vi "Windows.vi"(2 "Tau":dbl[](array[numeric]) format="%.3f", 3 "WINDOW":u16(ring) items=["FlatTop1", "FlatTop2", "FlatTop3", "FlatTop4", "FlatTop5", "FlatTop6"]) -> (0 "dPsi":dbl[](array[numeric]) format="%.3g", 1 "Psi":dbl[](array[numeric]) format="%.3g")   [LabVIEW 2022 SP3]
uses:
  <vilib>/Utility/file.llb/Read From Spreadsheet File (DBL).vi
  <vilib>/express/express arith-compare/Formula/XNode/ExpressFormulaBlockNode.xnode
panel:
  in  "ROWS":dbl
  in  "NEURONS":dbl
  in  "COLS":dbl
  in  "K":dbl
  out "DERIVATE FlatTop":dbl[][](array[numeric])
  out "FUNCTION FlatTop":dbl[][](array[numeric])
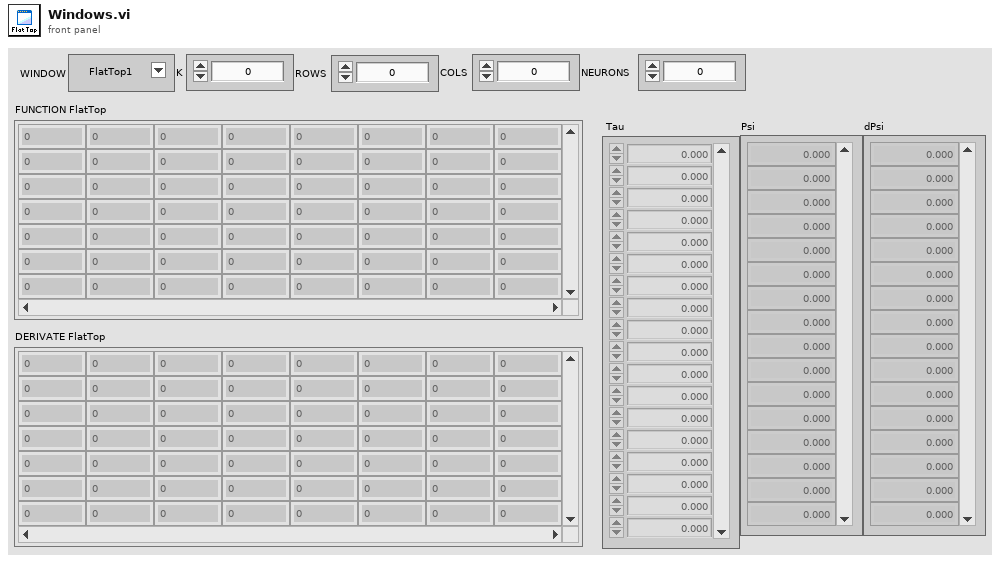
[diagram p1: front panel]
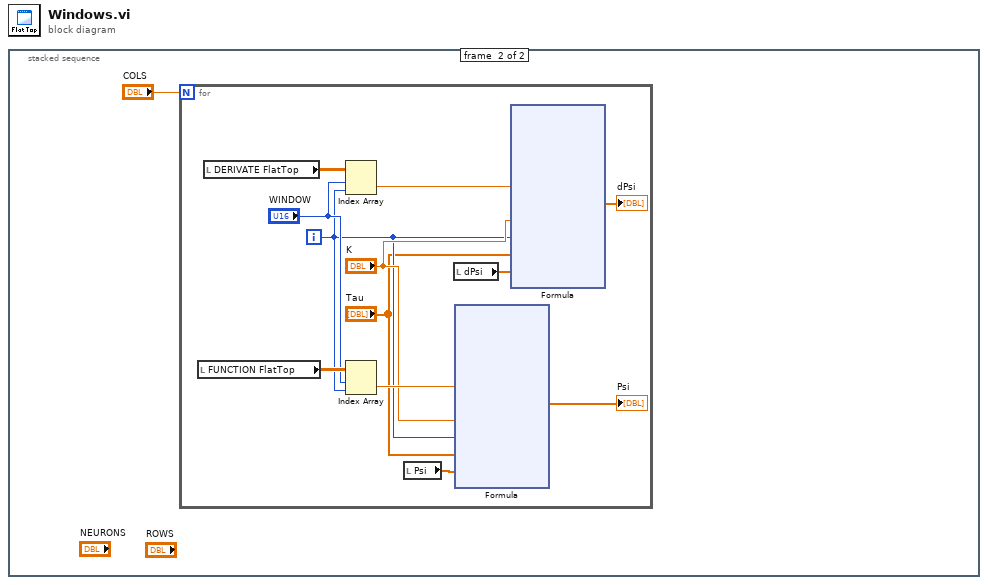
[diagram p0: block diagram]
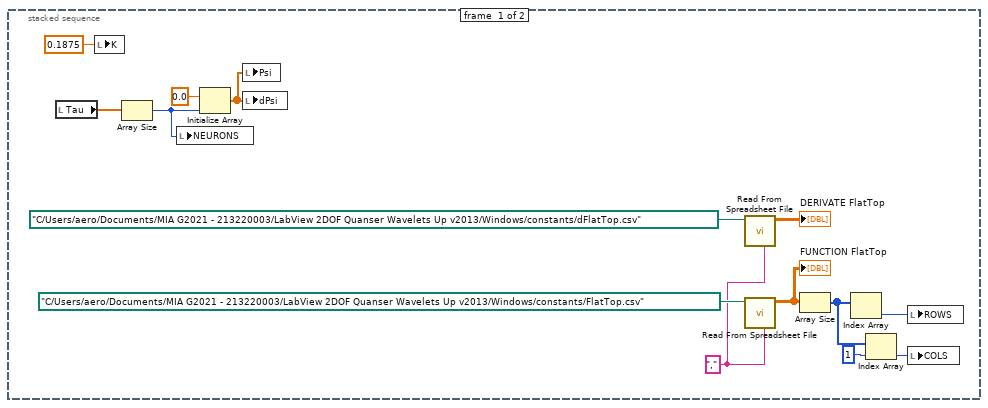
[diagram p2: hidden frame]
diagram:
  n1 = stacked-sequence {
    frame #0 {
      w2 = "," ("delimiter (\\t)")
      n2 = local read "Tau"() -> (w9:dbl[])
      n3 = local write "K"(0.1875 ("K")) -> ()
      n4 = Array Size(array=w9) -> (size(s)=w7:i32)
      n5 = local write "NEURONS"(w7) -> ()
      n6 = Initialize Array(0.0 ("element"), w7) -> (w6:dbl[])
      n7 = local write "Psi"(w6) -> ()
      n8 = local write "dPsi"(w6) -> ()
      n9 = call-poly <vilib>:"Read From Spreadsheet File.vi"("delimiter (\\t)"=w2, "file path (dialog if empty)"=path "C:/Users/aero/Documents/MIA G2021 - 213220003/LabView 2DOF Quanser Wavelets Up v2013/Windows/constants/dFlatTop.csv") -> ("all rows"=→"DERIVATE FlatTop":dbl[][])  [unwired: 5 in, 4 out]
      n10 = call-poly <vilib>:"Read From Spreadsheet File.vi"("delimiter (\\t)"=w2, "file path (dialog if empty)"=path "C:/Users/aero/Documents/MIA G2021 - 213220003/LabView 2DOF Quanser Wavelets Up v2013/Windows/constants/FlatTop.csv") -> ("all rows"=w4:dbl[][])  [unwired: 5 in, 4 out]
      "FUNCTION FlatTop" <- w4
      n11 = Array Size(array=w4) -> (size(s)=w12:i32[])
      n12 = Index Array(array=w12) -> (element=w13:i32)  [unwired: 1 in]
      n13 = Index Array(array=w12, index=1) -> (element=w10:i32)
      n14 = local write "ROWS"(w13) -> ()
      n15 = local write "COLS"(w10) -> ()
    }
    frame #1 {
      n16 = for {
        N: "COLS" -> [_]
        i -> [w19]
        n17 = local read "FUNCTION FlatTop"() -> (w27:dbl[][])
        n18 = local read "DERIVATE FlatTop"() -> (w22:dbl[][])
        n19 = Index Array(array=w22, index (row)="WINDOW", index (col)=w19) -> (element=w23:dbl)
        n20 = Index Array(array=w27, index (row)="WINDOW", index (col)=w19) -> (element=w26:dbl)
        n21 = local read "Psi"() -> (w24:dbl[])
        n22 = local read "dPsi"() -> (w16:dbl[])
        n23 = xnode "Formula"("A"=w26, "K"="K", "i"=w19, "tau"="Tau", "F"=w24) -> ("Result"=→"Psi":dbl[])  [unwired: 1 in, 1 out]
        n24 = xnode "Formula"("B"=w23, "K"="K", "i"=w19, "tau"="Tau", "dF"=w16) -> ("Result"=→"dPsi":dbl[])  [unwired: 1 in, 1 out]
      }
    }
  }
